vi "GOOP_ProviderClasses_Sorting.vi"(4 "ProvidersClassesActive":bool[](array[boolean]), 6 "ProvidersClassesSortOrder":string[](array[string]), 8 "error in (no error)":errorcluster, 10 "IgnoreFilter(False)":bool, 11 "AllClassProvidersIn(OriginalNames)":string[](array[string])) -> (0 "error out":errorcluster, 2 "AllClassProvidersActiveSettingOut":bool[](array[boolean]), 3 "AllClassProvidersOut(OriginalNames)":string[](array[string]))   [LabVIEW 2020]
uses:
  <vilib>/Utility/config.llb/Write Key (String).vi
  <vilib>/Utility/config.llb/Write Key (Boolean).vi
  <vilib>/Utility/config.llb/Read Key (String).vi
  <vilib>/Utility/config.llb/Read Key (Boolean).vi
  <vilib>/Utility/config.llb/NI_LVConfig.lvlib
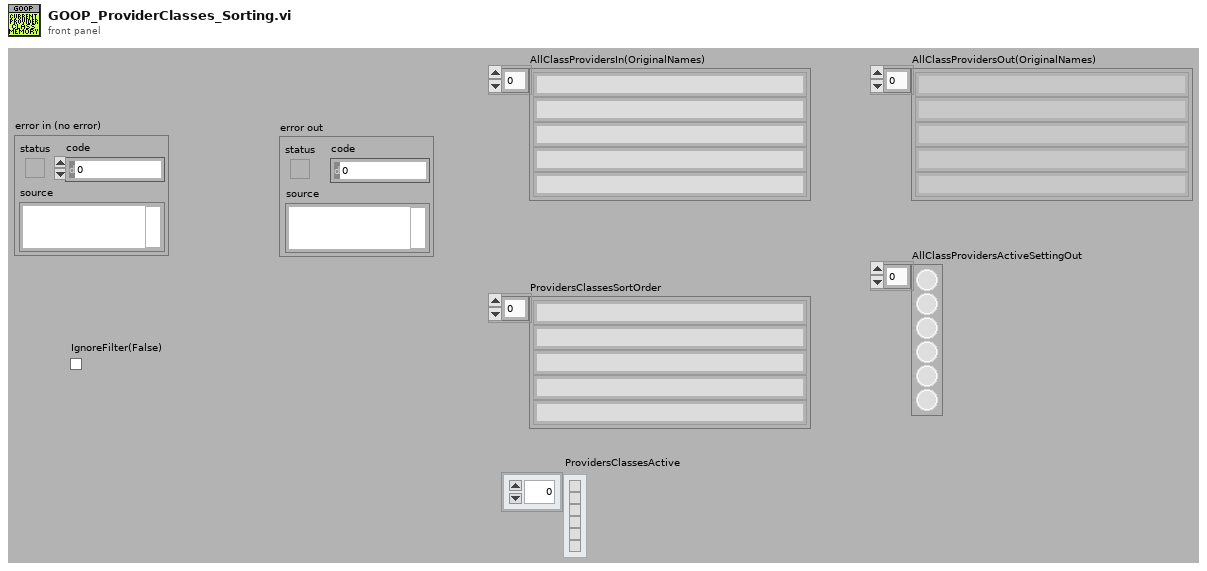
[diagram p1: front panel]
types:
  T1 = typedef "NI_LVConfig.lvlib/Config Data RefNum.ctl" = refnum<k1>
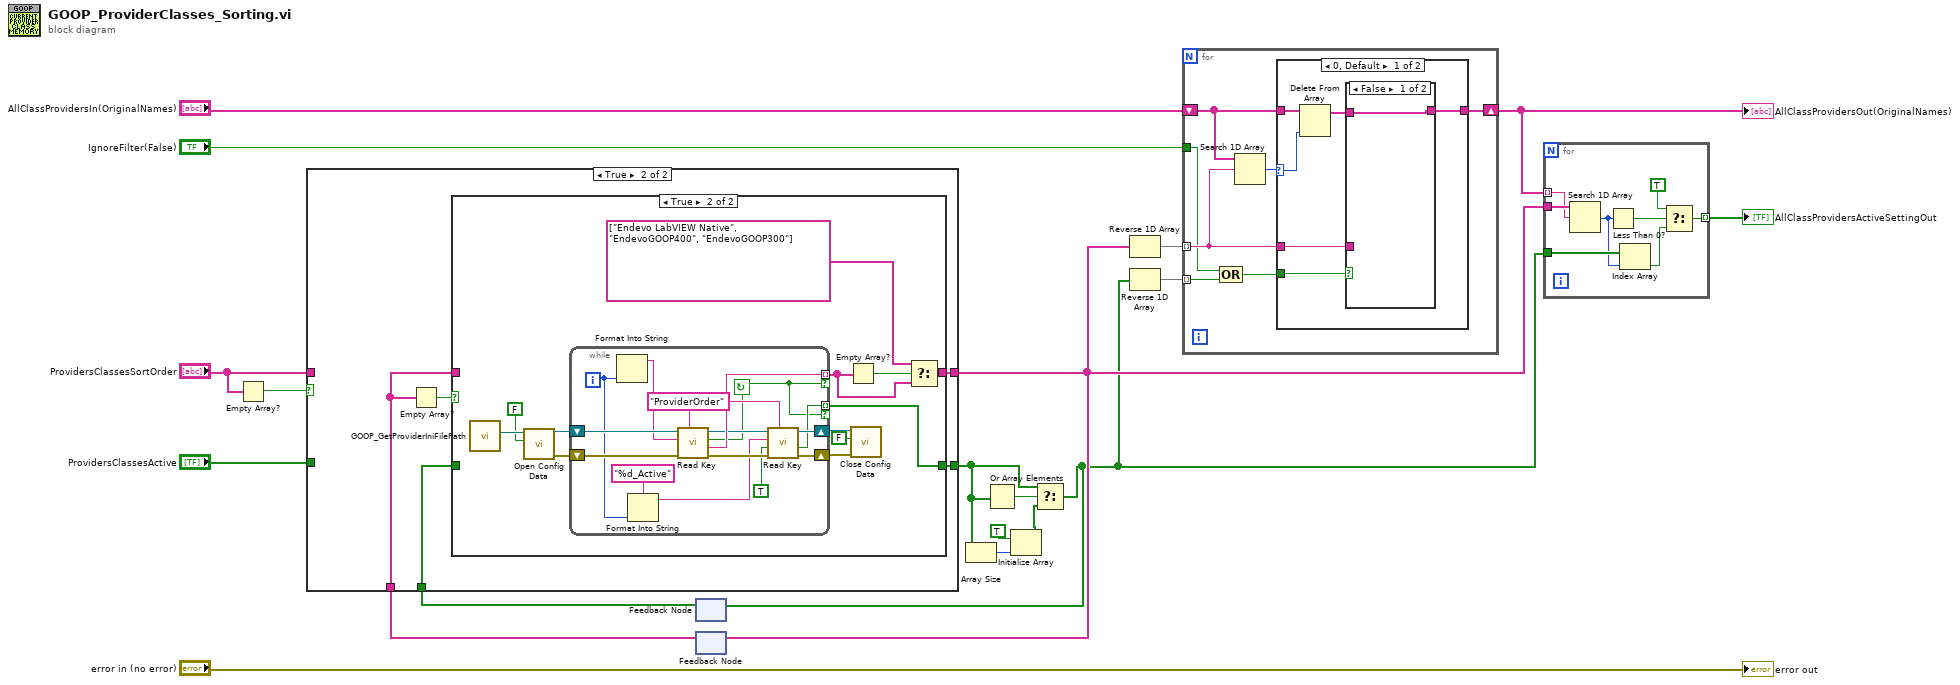
[diagram p0: block diagram]
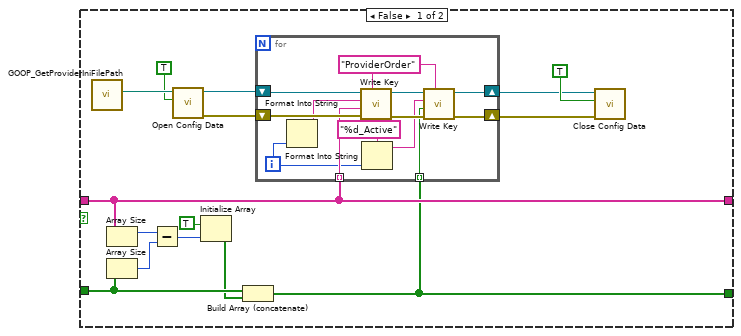
[diagram p2: hidden frame]
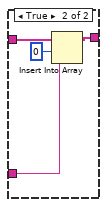
[diagram p4: hidden frame]
diagram:
  n1 = Empty Array?(array="ProvidersClassesSortOrder") -> (empty?=w15:bool)
  n2 = feedback #1() -> (w11:bool[])  [unwired: 1 in]
  n3 = feedback #2() -> (w18:string[])  [unwired: 1 in]
  n4 = case shown="True" w15 {
    tunnel: w18 -> [_ w51]
    tunnel: [w27 w50] -> w9
    tunnel: "ProvidersClassesSortOrder" -> [w27 _]
    tunnel: "ProvidersClassesActive" -> [w22 _]
    tunnel: [w20 w49] -> w2
    tunnel: w11 -> [_ w48]
    frame False {
      n5 = call <resource>:"GOOP_GetProviderIniFilePath.vi"() -> ("ProviderIniPath"=w34:path)  [unwired: 10 in, 1 out]
      n6 = Array Size(array=w27) -> (size(s)=w26:i32)
      n7 = Array Size(array=w22) -> (size(s)=w25:i32)
      n8 = Subtract(x=w26, y=w25) -> (x-y=w24:i32)
      n9 = call <vilib>:"Open Config Data.vi"("create file if necessary (T)"=TRUE ("create file if necessary? (T)"), "configuration file path"=w34) -> ("error out"=w30:errorcluster, "refnum"=w31:T1)  [unwired: 7 in, 1 out]
      n10 = Initialize Array(TRUE ("create file if necessary? (T)"), w24) -> (w21:bool[])
      n11 = Build Array (concatenate)(w22, w21) -> (w20:bool[])
      n12 = for {
        shift-right: [w42] -> w28
        shift-left: w31 -> [w47]
        shift-right: [w40] -> w29
        shift-left: w30 -> [w46]
        tunnel: w27 -> [w44] mode=indexing
        tunnel: w20 -> [w36] mode=indexing
        i -> [w39]
        w35 = "ProviderOrder" ("section")
        n13 = Format Into String(w39) -> (resulting string=w45:string)  [unwired: 3 in, 1 out]
        n14 = call-poly <vilib>:"Write Key.vi"("section"=w35, "error in (no error)"=w46, "value"=w44, "key"=w45, "refnum"=w47) -> ("error out"=w41:errorcluster, "refnum out"=w43:T1)  [unwired: 4 in, 1 out]
        n15 = Format Into String(format string="%d_Active", w39) -> (resulting string=w37:string)  [unwired: 2 in, 1 out]
        n16 = call-poly <vilib>:"Write Key.vi"("section"=w35, "error in (no error)"=w41, "value"=w36, "key"=w37, "refnum"=w43) -> ("error out"=w40:errorcluster, "refnum out"=w42:T1)  [unwired: 4 in, 1 out]
      }
      n17 = call <vilib>:"Close Config Data.vi"("error in (no error)"=w29, "write file if changed (T)"=TRUE, "refnum"=w28) -> ()  [unwired: 7 in, 2 out]
    }
    frame True {
      n18 = Empty Array?(array=w51) -> (empty?=w52:bool)
      n19 = case shown="True" w52 {
        tunnel: [w54 w56] -> w50
        tunnel: w51 -> [w54 _]
        tunnel: [w53 w55] -> w49
        tunnel: w48 -> [w53 _]
        frame False {
        }
        frame True {
          n20 = call <resource>:"GOOP_GetProviderIniFilePath.vi"() -> ("ProviderIniPath"=w66:path)  [unwired: 10 in, 1 out]
          n21 = call <vilib>:"Open Config Data.vi"("create file if necessary (T)"=FALSE ("create file if necessary? (T)"), "configuration file path"=w66) -> ("error out"=w64:errorcluster, "refnum"=w63:T1)  [unwired: 7 in, 1 out]
          n22 = while {
            shift-right: [w72] -> w62
            shift-left: w64 -> [w81]
            shift-right: [w73] -> w61
            shift-left: w63 -> [w80]
            tunnel: [w78] -> w57 mode=indexing if=w67
            tunnel: [w68] -> w55 mode=indexing if=w67
            i -> [w77]
            stop <- w67 continue-if-true
            w71 = "ProviderOrder" ("section")
            n23 = Format Into String(w77) -> (resulting string=w79:string)  [unwired: 3 in, 1 out]
            n24 = Format Into String(format string="%d_Active", w77) -> (resulting string=w70:string)  [unwired: 2 in, 1 out]
            n25 = call-poly <vilib>:"Read Key.vi"("section"=w71, "error in (no error)"=w81, "key"=w79, "refnum"=w80) -> ("error out"=w74:errorcluster, "value"=w78:string, "found?"=w67:bool, "refnum out"=w75:T1)  [unwired: 4 in]
            n26 = call-poly <vilib>:"Read Key.vi"("section"=w71, "error in (no error)"=w74, "default value"=TRUE, "key"=w70, "refnum"=w75) -> ("error out"=w72:errorcluster, "value"=w68:bool, "refnum out"=w73:T1)  [unwired: 3 in, 1 out]
          }
          n27 = Empty Array?(array=w57) -> (empty?=w59:bool)
          n28 = call <vilib>:"Close Config Data.vi"("error in (no error)"=w62, "write file if changed (T)"=FALSE, "refnum"=w61) -> ()  [unwired: 7 in, 2 out]
          n29 = Select(t=string[] ["Endevo LabVIEW Native", "EndevoGOOP400", "EndevoGOOP300"] ("AllClassProviders"), s=w59, f=w57) -> (s? t:f=w56:string[])
        }
      }
    }
  }
  n30 = feedback-in #2(w9) -> ()
  n31 = Array Size(array=w2) -> (size(s)=w5:i32)
  n32 = Or Array Elements(Boolean array=w2) -> (logical OR=w6:bool)
  n33 = Initialize Array(TRUE, w5) -> (w4:bool[])
  n34 = Select(t=w2, s=w6, f=w4) -> (s? t:f=w1:bool[])
  n35 = feedback-in #1(w1) -> ()
  n36 = Reverse 1D Array(array=w9) -> (reversed array=w16:string[])
  n37 = Reverse 1D Array(array=w1) -> (reversed array=w12:bool[])
  n38 = for {
    shift-right: [w86] -> w10
    shift-left: "AllClassProvidersIn(OriginalNames)" -> [w87]
    tunnel: w16 -> [w85] mode=indexing
    tunnel: w12 -> [w84] mode=indexing
    tunnel: "IgnoreFilter(False)" -> [w82]
    n39 = Compound Arithmetic op=OR(w82, w84) -> (w83:bool)
    n40 = Search 1D Array(1D array=w87, element=w85) -> (index of element=w88:i32)  [unwired: 1 in]
    n41 = case shown="0, Default" w88 {
      selector: w88 -> [w93 _]
      tunnel: w87 -> [w94 w100]
      tunnel: [w90 w100] -> w86
      tunnel: w85 -> [w91 _]
      tunnel: w83 -> [w89 _]
      frame 0, Default {
        n42 = Delete From Array(array=w94, index=w93) -> (array with subset deleted=w92:string[])  [unwired: 1 in, 1 out]
        n43 = case shown="False" w89 {
          tunnel: w92 -> [w95 w99]
          tunnel: w91 -> [_ w98]
          tunnel: [w95 w96] -> w90
          frame False {
          }
          frame True {
            n44 = Insert Into Array(array=w99, index=0, new element=w98) -> (w96:string[])
          }
        }
      }
      frame -1 {
      }
    }
  }
  "AllClassProvidersOut(OriginalNames)" <- w10
  n45 = for {
    tunnel: w10 -> [w107] mode=indexing
    tunnel: w9 -> [w108]
    tunnel: w1 -> [w104]
    tunnel: [w101] -> w7 mode=indexing
    n46 = Search 1D Array(1D array=w108, element=w107) -> (index of element=w103:i32)  [unwired: 1 in]
    n47 = Less Than 0?(x=w103) -> (x < 0?=w106:bool)
    n48 = Index Array(array=w104, index=w103) -> (element=w102:bool)
    n49 = Select(t=TRUE, s=w106, f=w102) -> (s? t:f=w101:bool)
  }
  "AllClassProvidersActiveSettingOut" <- w7
  "error out" <- "error in (no error)"
